vi "Stop Core.vi"(10 "final error code":i32, 11 "Connection Listener in":refnum<class "Connection Listener.lvclass">) -> (3 "Connection Listener out":refnum<class "Connection Listener.lvclass">)   [LabVIEW 2017, in "Connection Listener.lvlib" / "Connection Listener.lvclass"]
doc: "(<B>Filename</B>: Actor Framework.lvlib:Actor.lvclass:Stop Core.vi)\n\nDefines what the actor does before it stops. Use the <B>final error code</B> input to determine whether the actor shut down in response to an error.\n\nBy default, this method does nothing. A descendant class may override it to define behavior, such as shutting down any processes the actor initiated in its override of the Actor Core method."
uses:
  Connection Listener.lvclass
  Connection Listener.lvclass/Connection Listener.ctl
  <vilib>/ActorFramework/Message Enqueuer/Message Enqueuer.lvclass/Message Enqueuer.ctl
  <vilib>/ActorFramework/Message Enqueuer/Enqueue.vi
  <vilib>/ActorFramework/Stop Msg/Stop Msg.lvclass
  Applications/National Instruments/LabVIEW 2017 64-bit/vi.lib/ActorFramework/Message/Message.lvclass
  <vilib>/ActorFramework/Message Priority Queue/Priority Enqueue.vi
  Actor wHelper/Actor wHelper/Actor wHelper.lvclass
  <vilib>/MediaMongrels Ltd/WebSockets/Sockets/VISA TCP Listener/VISA TCP Listener.lvclass
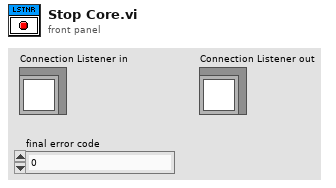
[diagram p1: front panel]
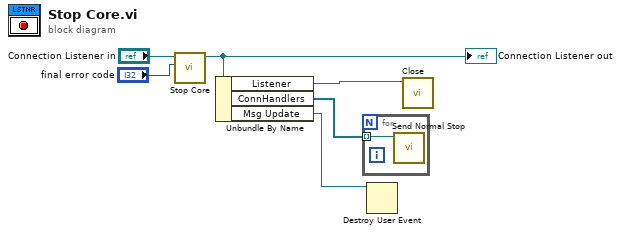
[diagram p0: block diagram]
diagram:
  n1 = call-parent "Stop Core.vi"("final error code"="final error code", "Actor wHelper in"="Connection Listener in") -> ("Actor wHelper out"=w4:refnum<class "Connection Listener.lvclass">)  [unwired: 9 in]
  "Connection Listener out" <- w4
  n2 = Unbundle By Name(w4) -> ("Listener"=w3:refnum<class "VISA TCP Listener.lvclass">, "ConnHandlers"=w2:refnum<class "Message Enqueuer.lvclass">[], "Msg Update"=w1:refnum<user-event>)
  n3 = for {
    tunnel: w2 -> [w7] mode=indexing
    n4 = call <vilib>:"Send Normal Stop.vi"("Message Enqueuer"=w7) -> ()  [unwired: 10 in, 1 out]
  }
  n5 = Destroy User Event(user event=w1) -> ()  [unwired: 1 in, 1 out]
  n6 = call-dynamic "Close.vi"("VISA TCP Listener in"=w3) -> ()  [unwired: 10 in, 1 out]
